vi "Create.vi"(8 "error in (no error)":errorcluster) -> (0 "error out":errorcluster, 3 "Event Registration Refnum":refnum<event-registration>)   [LabVIEW 2020, in "WebServiceImporter.lvlib" / "Main Panel.lvlib" / "Input WSDL.lvlib" / "Events.lvlib"]
uses:
  <vilib>/Platform/WebService/Main Panel/Pages/Input WSDL/Events/Events.lvlib
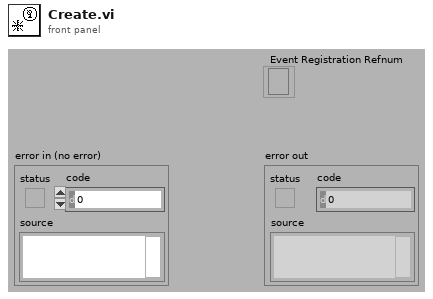
[diagram p1: front panel]
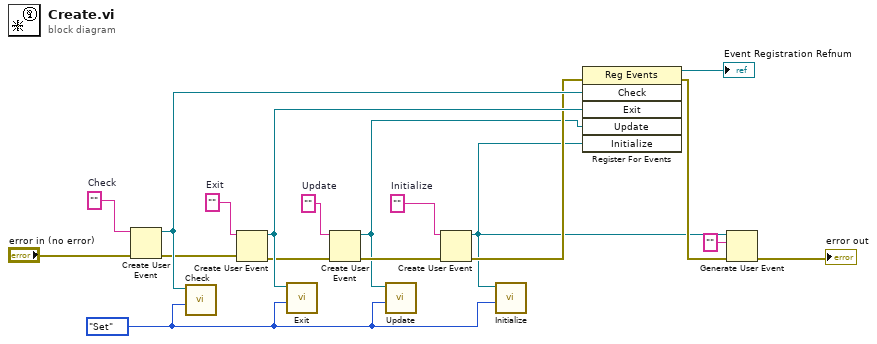
[diagram p0: block diagram]
diagram:
  w5 = ""  # Update
  w13 = ""  # Initialize
  w15 = ""  # Exit
  w3 = enum16{"Get", "Set"}."Set" ("Operation")
  w17 = ""  # Check
  n1 = Create User Event(user event datatype=w17, error in="error in (no error)") -> (user event=w16:refnum<user-event>, error out=w14:errorcluster)
  n2 = call <vilib>:"Check.vi"("Operation"=w3, "user event"=w16) -> ()  [unwired: 8 in, 2 out]
  n3 = Create User Event(user event datatype=w15, error in=w14) -> (user event=w12:refnum<user-event>, error out=w6:errorcluster)
  n4 = call <vilib>:"Exit.vi"("Operation"=w3, "user event"=w12) -> ()  [unwired: 8 in, 2 out]
  n5 = Create User Event(user event datatype=w5, error in=w6) -> (user event=w2:refnum<user-event>, error out=w4:errorcluster)
  n6 = call <vilib>:"Update.vi"("Operation"=w3, "user event"=w2) -> ()  [unwired: 8 in, 2 out]
  n7 = Create User Event(user event datatype=w13, error in=w4) -> (user event=w7:refnum<user-event>, error out=w11:errorcluster)
  n8 = call <vilib>:"Initialize.vi"("Operation"=w3, "user event"=w7) -> ()  [unwired: 9 in, 1 out]
  n9 = register-events(error in=w11, w16, w12, w2, w7) -> (reference out=→"Event Registration Refnum":refnum<event-registration>, error out=w9:errorcluster)  [unwired: 1 in]
  n10 = Generate User Event(user event=w7, event data cluster="" ("event data"), error in=w9) -> (error out=→"error out":errorcluster)  [unwired: 1 in, 1 out]
